vi "Reverse Drive Option.vi"(2 "Y-Value":dbl, 3 "X-Value":dbl, 4 "Reverse?":bool) -> (0 "Y Drive Values":dbl, 1 "X Drive Values":dbl)   [LabVIEW 2013]
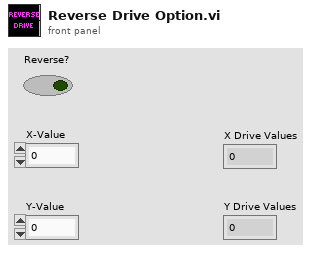
[diagram p1: front panel]
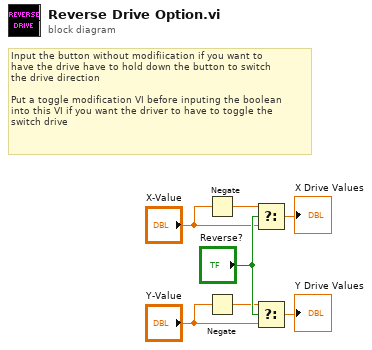
[diagram p0: block diagram]
diagram:
  # "Input the button without modifiication if you want to\nhave the drive have to hold down the button to switch\nthe drive direction\n\nPut a toggle modification VI before inputing the boolean\ninto this VI if you want the driver to have to toggle the\nswitch drive"
  n1 = Negate(x="X-Value") -> (-x=w5:dbl)
  n2 = Negate(x="Y-Value") -> (-x=w3:dbl)
  n3 = Select(t=w5, s="Reverse?", f="X-Value") -> (s? t:f=→"X Drive Values":dbl)
  n4 = Select(t=w3, s="Reverse?", f="Y-Value") -> (s? t:f=→"Y Drive Values":dbl)
